vi "SUBVI_decode_image.vi"(10 "Numeric":dbl, 11 "String in":string) -> (3 "String out":string)   [LabVIEW 2021]
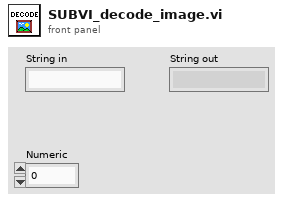
[diagram p1: front panel]
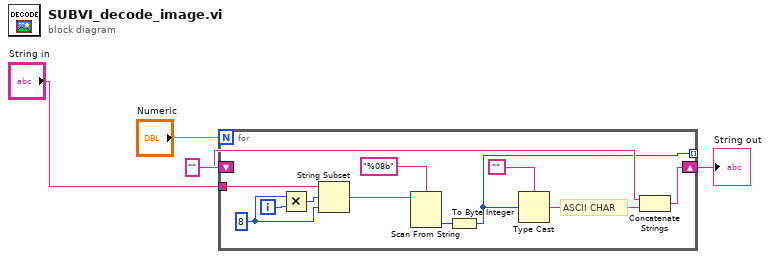
[diagram p0: block diagram]
diagram:
  n1 = for {
    N: "Numeric" -> [_]
    tunnel: "String in" -> [w16]
    shift-right: [w6] -> w2
    shift-left: "" -> [w8]
    tunnel: [w5] -> _ mode=indexing
    i -> [w15]
    w14 = 8 ("length (rest)")
    # "ASCII CHAR"
    n2 = Multiply(x=w14, y=w15) -> (x*y=w13:i32)
    n3 = String Subset(string=w16, offset (0)=w13, length (rest)=w14) -> (substring=w9:string)
    n4 = Scan From String(format string="%08b", input string=w9) -> (output 1=w10:i32)  [unwired: 3 in, 3 out]
    n5 = To Byte Integer(number=w10) -> (8bit integer=w5:i8)
    n6 = Type Cast(type="", x=w5) -> (*(type *) &x=w7:string)
    n7 = Concatenate Strings(w8, w7) -> (w6:string)
  }
  "String out" <- w2
